vi "Stepper Drive Publish Event Loop Exit.vi"(8 "error in (no error)":errorcluster, 11 "Axis Config Constant":T1) -> ()   [LabVIEW 2016, in "SMD-7615.lvlib"]
uses:
  SMD-7615.lvlib
  CTL/Stepper Drive Config.ctl
  CTL/SV General.ctl
  CTL/SV Inputs.ctl
  CTL/SV Outputs.ctl
  LUL-All/LUL-Syslog/LUL-SysLog.lvlib
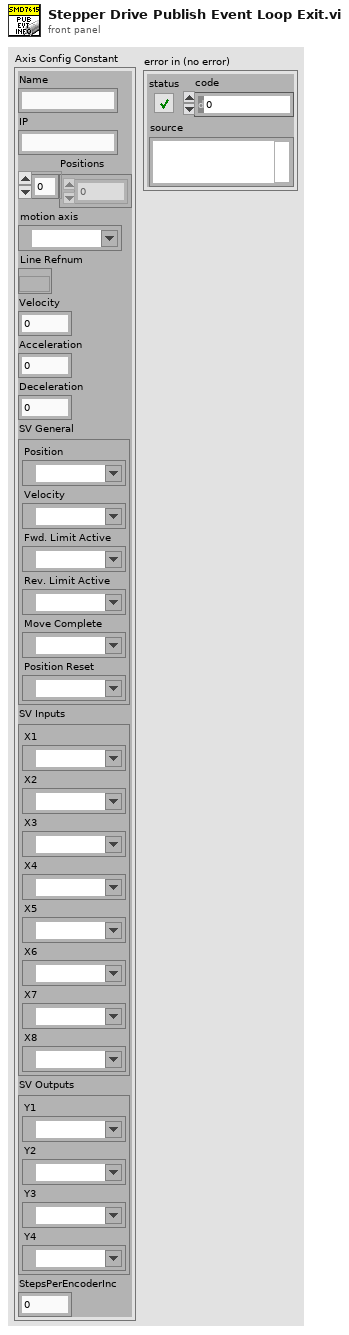
[diagram p1: front panel]
types:
  T1 = typedef "SMD-7615.lvlib/Stepper Drive Config.ctl" = cluster{"Name":string, "IP":string, "Positions":dbl[], "motion axis ":refnum<k21>, "Line Refnum":refnum<k20>, "Velocity":dbl, "Acceleration":dbl, "Deceleration":dbl, "SV General":T2, "SV Inputs":T3, "SV Outputs":T4, "StepsPerEncoderInc":i32}
  T2 = typedef "SMD-7615.lvlib/SV General.ctl" = cluster{"Position":refnum<k21>, "Velocity":refnum<k21>, "Fwd. Limit Active":refnum<k21>, "Rev. Limit Active":refnum<k21>, "Move Complete":refnum<k21>, "Position Reset":refnum<k21>}
  T3 = typedef "SMD-7615.lvlib/SV Inputs.ctl" = cluster{"X1":refnum<k21>, "X2":refnum<k21>, "X3":refnum<k21>, "X4":refnum<k21>, "X5":refnum<k21>, "X6":refnum<k21>, "X7":refnum<k21>, "X8":refnum<k21>}
  T4 = typedef "SMD-7615.lvlib/SV Outputs.ctl" = cluster{"Y1":refnum<k21>, "Y2":refnum<k21>, "Y3":refnum<k21>, "Y4":refnum<k21>}
  T5 = typedef "LUL-SysLog.lvlib/SysLog Severity.ctl" = enum16{"Emergency", "Alert", "Critical", "Error", "Wanring", "Notice", "Informational", "Debug"}
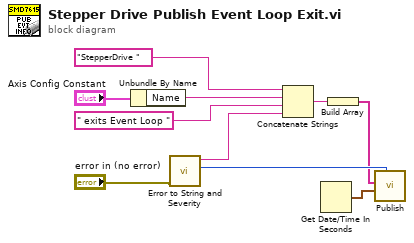
[diagram p0: block diagram]
diagram:
  n1 = Unbundle By Name("Axis Config Constant") -> ("Name"=w9:string)
  n2 = call "Error to String and Severity.vi"("error in (no error)"="error in (no error)") -> ("Severity"=w3:T5, "Error Text"=w4:string)  [unwired: 9 in]
  n3 = Concatenate Strings("StepperDrive " ("string"), w9, " exits Event Loop " ("string"), w4) -> (w2:string)
  n4 = Get Date/Time In Seconds() -> (seconds since 1Jan1904=w8:timestamp)
  n5 = Build Array(w2) -> (w1:string[])
  n6 = call "Publish.vi"("Severity"=w3, "current time"=w8, "Message"=w1) -> ()  [unwired: 8 in, 1 out]
